vi "DSF.Engine.Memory.Buffer.Set Buffer Config.vi"(8 "error in (no error)":errorcluster, 10 "Buffer Config":refnum<class "DSF.Memory.Buffer.Config.lvclass">, 11 "Buffer in":refnum<class "DSF.Engine.Memory.Buffer.lvclass">) -> (0 "error out":errorcluster, 3 "Buffer out":refnum<class "DSF.Engine.Memory.Buffer.lvclass">)   [LabVIEW 2016, in "DSF.Engine.lvlib" / "DSF.Engine.Memory.Buffer.lvclass"]
uses:
  DSF.Engine.Memory.Buffer.lvclass
  DSF.Memory.Buffer.Config.lvclass
  DSF.Engine.Memory.Buffer.lvclass/DSF.Engine.Memory.Buffer.ctl
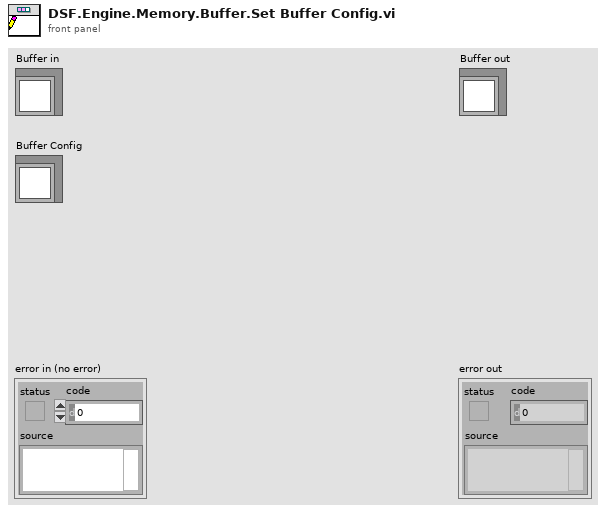
[diagram p1: front panel]
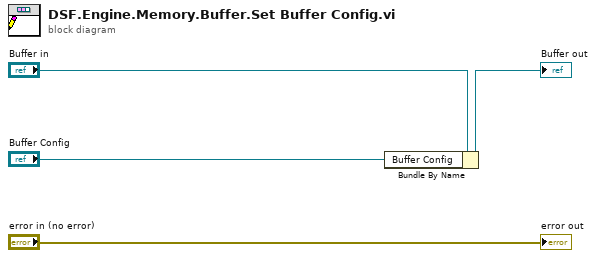
[diagram p0: block diagram]
diagram:
  n1 = Bundle By Name(cluster="Buffer in", "Buffer Config"="Buffer Config") -> (→"Buffer out":refnum<class "DSF.Engine.Memory.Buffer.lvclass">)
  "error out" <- "error in (no error)"
